vi "poly_control_ref_from_name_single.vi"(8 "error in (no error)":errorcluster, 9 "control name":string, 10 "vi ref":refnum<vi>) -> (0 "error out":errorcluster, 1 "ctrl ref":refnum<vi>, 2 "vi ref dup":refnum<vi>, 4 "found?":bool)   [LabVIEW 2015, in "_ref_tools_polys.lvlib"]
uses:
  _ref_tools_polys.lvlib
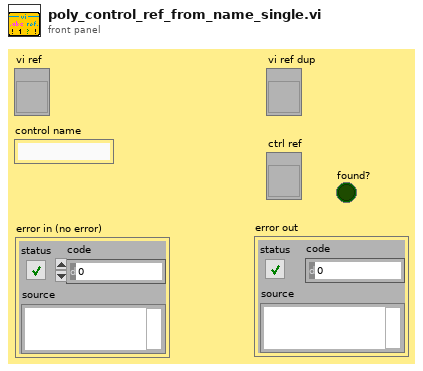
[diagram p1: front panel]
types:
  T1 = cluster{"control name":string, "vi ref":refnum<vi>, "ctrl ref":refnum<vi>, "found?":bool}
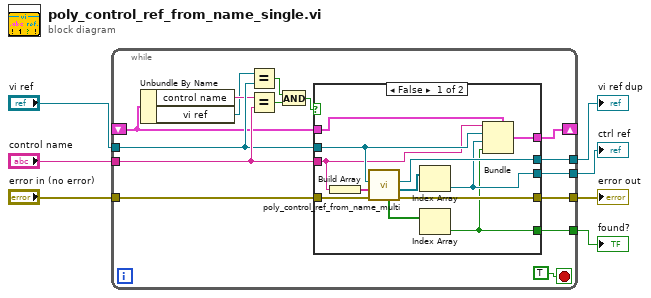
[diagram p0: block diagram]
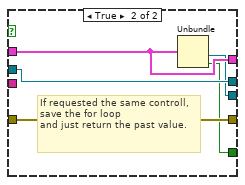
[diagram p2: hidden frame]
diagram:
  n1 = while {
    tunnel: [w20] -> w5
    tunnel: "control name" -> [w13]
    tunnel: "vi ref" -> [w12]
    tunnel: "error in (no error)" -> [w15]
    shift-right: [w11] -> _
    shift-left: _ -> [w8]
    tunnel: [w21] -> w6
    tunnel: [w14] -> w1
    tunnel: [w22] -> w7
    stop <- TRUE stop-if-true
    n2 = Unbundle By Name(w8) -> ("control name"=w10:string, "vi ref"=w9:refnum<vi>)
    n3 = Equal?(x=w9, y=w12) -> (x = y?=w19:bool)
    n4 = Equal?(x=w10, y=w13) -> (x = y?=w18:bool)
    n5 = And(x=w19, y=w18) -> (x .and. y?=w17:bool)
    n6 = case shown="False" w17 {
      tunnel: w12 -> [w32 w38]
      tunnel: [w27 w36] -> w21
      tunnel: [w25 w39] -> w20
      tunnel: w15 -> [w24 w39]
      tunnel: [w29 w38] -> w22
      tunnel: [w23 w35] -> w14
      tunnel: w13 -> [w31 _]
      tunnel: [w34 w37] -> w11
      tunnel: w8 -> [w33 w37]
      frame False {
        n7 = Build Array(w31) -> (w30:string[])
        n8 = call "poly_control_ref_from_name_multi.vi"("error in (no error)"=w24, "control names"=w30, "vi ref"=w32) -> ("error out"=w25:errorcluster, "ctrl refs"=w28:refnum<vi>[], "vi ref dup"=w29:refnum<vi>, "found?"=w26:bool[])  [unwired: 5 in]
        n9 = Index Array(array=w28) -> (element=w27:refnum<vi>)  [unwired: 1 in]
        n10 = Index Array(array=w26) -> (element=w23:bool)  [unwired: 1 in]
        n11 = Bundle(cluster=w33, "control name"=w31, "vi ref"=w32, "ctrl ref"=w27, "found?"=w23) -> (w34:T1)
      }
      frame True {
        # "If requested the same controll, save the for loop\nand just return the past value."
        n12 = Unbundle(w37) -> ("ctrl ref"=w36:refnum<vi>, "found?"=w35:bool)  [unwired: 2 out]
      }
    }
  }
  "vi ref dup" <- w7
  "ctrl ref" <- w6
  "error out" <- w5
  "found?" <- w1
